vi "车速实时记录系统.vi"() -> ()   [LabVIEW 2018]
panel:
  out "车速实时显示":dbl[](graph)
  in  "警示":string
  in  "停止":bool
  out "超速警告":bool
  out "时速":dbl(knob) scale=0.0..100.0
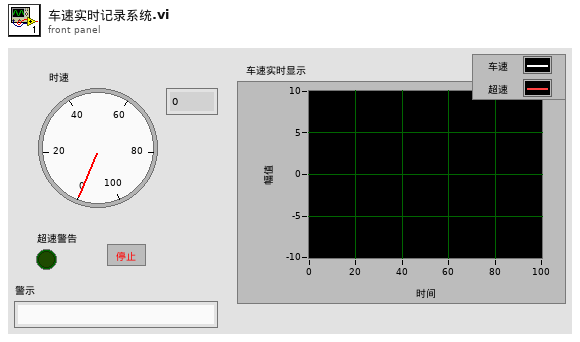
[diagram p1: front panel]
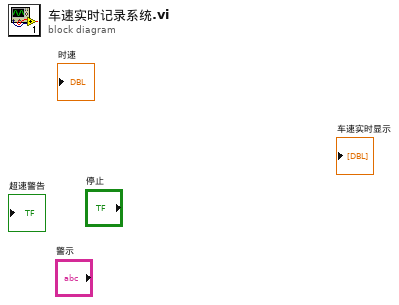
[diagram p0: block diagram]
diagram:
